vi "SLT Get Process Name.vi"(0 "handle":i32, 11 "error in (no error)":errorcluster) -> (4 "handle out":i32, 8 "ImageFileName":string, 15 "error out":errorcluster)   [LabVIEW 2013, in "ProcessInfo.lvlib"]
doc: "Retrieves the name of the executable file for the specified process."
uses:
  ProcessInfo.lvlib
  psapi.dll
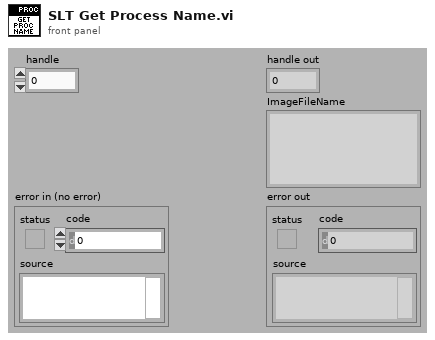
[diagram p1: front panel]
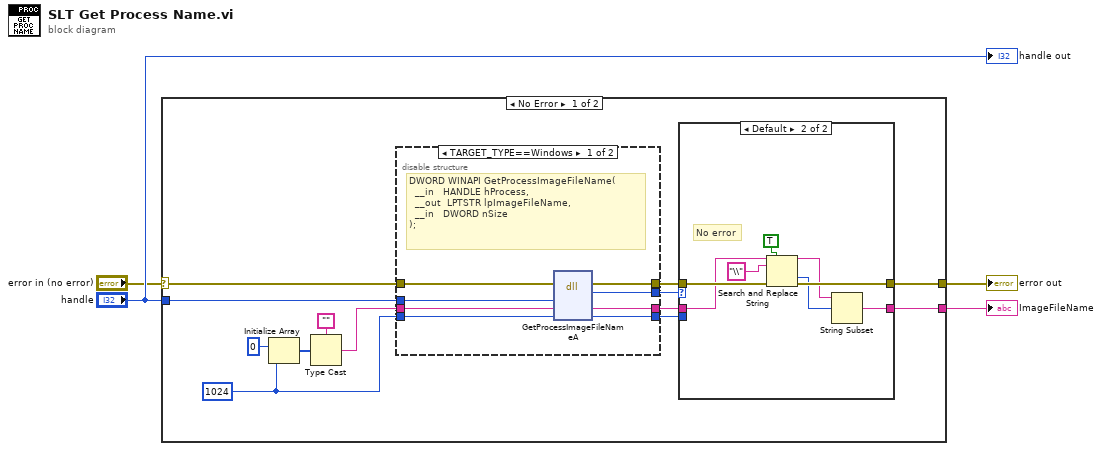
[diagram p0: block diagram]
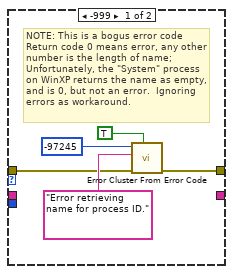
[diagram p3: hidden frame]
diagram:
  n1 = case shown="No Error" "error in (no error)" {
    selector: "error in (no error)" -> [w15 w43]
    tunnel: [w17 w43] -> w4
    tunnel: "handle" -> [w16 _]
    tunnel: [w13 _] -> w1
    frame No Error {
      w14 = u32 1024 ("Size")
      n2 = Initialize Array(u8 0 ("element"), w14) -> (w11:u8[])
      n3 = Type Cast(type="" ("pointerTostring"), x=w11) -> (*(type *) &x=w9:string)
      n4 = disable-structure shown="TARGET_TYPE==Windows" {
        disable-tunnel: w16 -> [w25 w28]
        disable-tunnel: w15 -> [w24 w29]
        disable-tunnel: w14 -> [w23 w26]
        disable-tunnel: w9 -> [w22 w27]
        disable-tunnel: [w21 w26] -> w8
        disable-tunnel: [w20 w28] -> w7
        disable-tunnel: [w19 w29] -> w6
        disable-tunnel: [w18 w27] -> w5
        frame condition #0 (active) {
          # "DWORD WINAPI GetProcessImageFileName(\n  __in   HANDLE hProcess,\n  __out  LPTSTR lpImageFileName,\n  __in   DWORD nSize\n);"
          n5 = dll-call lib="psapi.dll" fn="GetProcessImageFileNameA"(error in=w24, "handle"=w25, "ImageFileName"=w22, "Size"=w23) -> (error out=w19:errorcluster, "error"=w20:i32, "ImageFileName"=w18:string, "Size"=w21:u32)  [unwired: 3 in, 1 out]
        }
        frame condition #1 {
        }
      }
      n6 = case shown="Default" w7 {
        tunnel: w8 -> [_ _]
        tunnel: w6 -> [w30 w38]
        tunnel: [w31 w42] -> w17
        tunnel: w5 -> [_ w37]
        tunnel: [_ w36] -> w13
        frame -999 {
          # "NOTE: This is a bogus error code\nReturn code 0 means error, any other number is the length of name; Unfortunately, the \"System\" process on WinXP returns the name as empty, and is 0, but not an error.  Ignoring errors as workaround."
          n7 = call <vilib>:"Error Cluster From Error Code.vi"("show call chain? (False)"=TRUE, "error in (no error)"=w30, "error message (\"\")"="Error retrieving name for process ID." ("error message (\"\")"), "error code (0)"=-97245) -> ("error out"=w31:errorcluster)  [unwired: 5 in]
        }
        frame Default {
          # "No error"
          n8 = Search and Replace String(replace all?=TRUE ("replace all? (F)"), input string=w37, search string="\\", error in=w38) -> (result string=w41:string, offset past replacement=w35:i32, error out=w42:errorcluster)  [unwired: 5 out]
          n9 = String Subset(string=w41, offset (0)=w35) -> (substring=w36:string)  [unwired: 1 out]
        }
      }
    }
    frame Error {
    }
  }
  "error out" <- w4
  "ImageFileName" <- w1
  "handle out" <- "handle"
